vi "Read Samples_ID.vi"(8 "error in (no error)":errorcluster, 11 "DB in":refnum<class "DB.lvclass">) -> (0 "error out":errorcluster, 2 "Samples_ID":i16[](array[numeric]), 3 "DB out":refnum<class "DB.lvclass">)   [LabVIEW 2020, in "DB.lvclass"]
uses:
  DB.lvclass
  DB.lvclass/DB.ctl
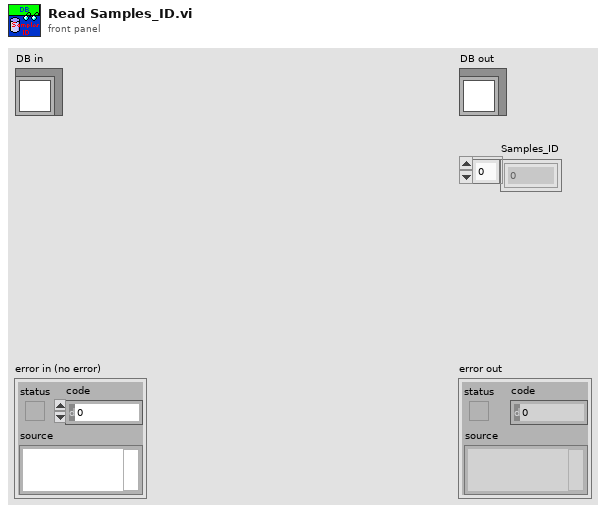
[diagram p1: front panel]
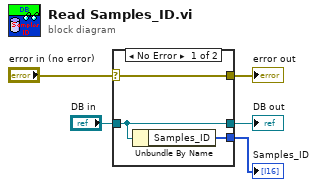
[diagram p0: block diagram]
diagram:
  n1 = case shown="No Error" "error in (no error)" {
    selector: "error in (no error)" -> [w8 w9]
    tunnel: [w8 w9] -> w4
    tunnel: [w7 w10] -> w2
    tunnel: "DB in" -> [w7 w10]
    tunnel: [w6 _] -> w1
    frame No Error {
      n2 = Unbundle By Name(w7) -> ("Samples_ID"=w6:i16[])
    }
    frame Error {
    }
  }
  "error out" <- w4
  "DB out" <- w2
  "Samples_ID" <- w1
